vi "SelectChip.vi"(8 "error in (no error)":errorcluster, 10 "chipSelection":string="LT9611", 11 "LT_UpgradeFlash in":refnum<class "LT_UpgradeFlash.lvclass">) -> (0 "error out":errorcluster, 1 "resultStr":string, 2 "ActionResult":bool, 3 "LT_UpgradeFlash out":refnum<class "LT_UpgradeFlash.lvclass">)   [LabVIEW 2017, in "LT_UpgradeFlash.lvclass"]
uses:
  LT_UpgradeFlash.lvclass
  D:/Project/Tymphany/LT_UpgradeFlash/LT_UpgradeFlash_dll/LT_UpgradeFlash_dll/bin/Debug/LT_UpgradeFlash_dll.dll
  LT_UpgradeFlash_dll/LT_UpgradeFlash_dll/bin/Debug/LT_UpgradeFlash_dll.dll
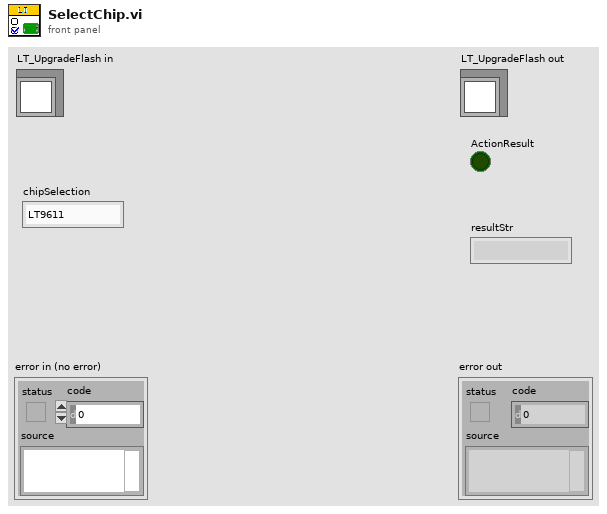
[diagram p1: front panel]
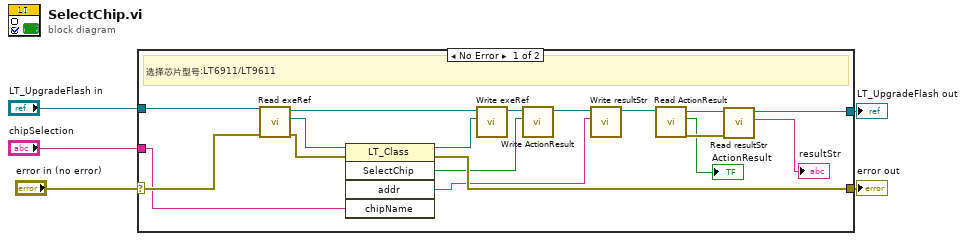
[diagram p0: block diagram]
diagram:
  n1 = case shown="No Error" "error in (no error)" {
    selector: "error in (no error)" -> [w16 w25]
    tunnel: [w22 w25] -> w4
    tunnel: [w11 w24] -> w2
    tunnel: "LT_UpgradeFlash in" -> [w7 w24]
    tunnel: "chipSelection" -> [w6 _]
    frame No Error {
      # "选择芯片型号:LT6911/LT9611"
      n2 = call-dynamic "Read exeRef.vi"("error in (no error)"=w16, "LT_UpgradeFlash in"=w7) -> ("error out"=w17:errorcluster, "exeRef"=w23:refnum<k24>, "LT_UpgradeFlash out"=w21:refnum<class "LT_UpgradeFlash.lvclass">)  [unwired: 7 in]
      n3 = invoke class="LT_Class" method="SelectChip"(reference=w23, error in=w17, "chipName"=w6) -> (reference out=w19:refnum<k24>, error out=w22:errorcluster, "SelectChip"=w18:bool, "addr"=w8:string)  [unwired: 2 in, 1 out]
      n4 = call-dynamic "Write exeRef.vi"("exeRef"=w19, "LT_UpgradeFlash in"=w21) -> ("LT_UpgradeFlash out"=w20:refnum<class "LT_UpgradeFlash.lvclass">)  [unwired: 8 in, 1 out]
      n5 = call-dynamic "Write ActionResult.vi"("ActionResult"=w18, "LT_UpgradeFlash in"=w20) -> ("LT_UpgradeFlash out"=w10:refnum<class "LT_UpgradeFlash.lvclass">)  [unwired: 8 in, 1 out]
      n6 = call-dynamic "Write resultStr.vi"("resultStr"=w8, "LT_UpgradeFlash in"=w10) -> ("LT_UpgradeFlash out"=w9:refnum<class "LT_UpgradeFlash.lvclass">)  [unwired: 8 in, 1 out]
      n7 = call-dynamic "Read ActionResult.vi"("LT_UpgradeFlash in"=w9) -> ("error out"=w14:errorcluster, "ActionResult"=→"ActionResult":bool, "LT_UpgradeFlash out"=w15:refnum<class "LT_UpgradeFlash.lvclass">)  [unwired: 8 in]
      n8 = call-dynamic "Read resultStr.vi"("error in (no error)"=w14, "LT_UpgradeFlash in"=w15) -> ("resultStr"=→"resultStr":string, "LT_UpgradeFlash out"=w11:refnum<class "LT_UpgradeFlash.lvclass">)  [unwired: 7 in, 1 out]
    }
    frame Error {
    }
  }
  "error out" <- w4
  "LT_UpgradeFlash out" <- w2
